vi "GetOtherStimulusArrayValues.vi"(3 "time between onset index":i32, 4 "fraction of time between index":i32, 5 "Cluster":cluster{"Value":sgl[][], "Value":i32[][]}, 6 "time since beginning of run":i32) -> (0 "time between onset index out":i32, 1 "fraction of time between index out":i32, 2 "stimulus settings":cluster{"outy3":sgl, "outy3":i32})   [LabVIEW 2015]
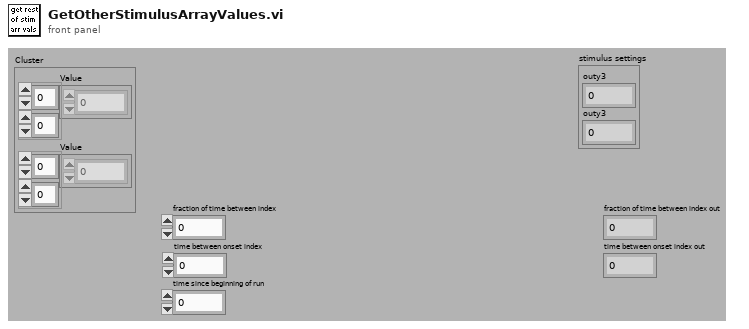
[diagram p1: front panel]
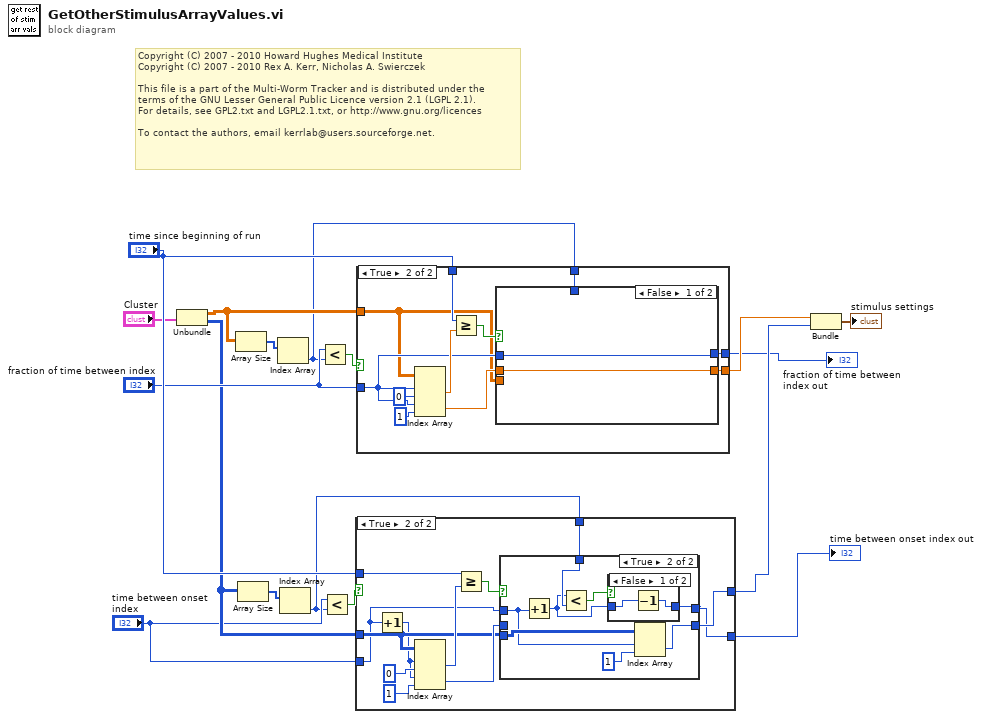
[diagram p0: block diagram]
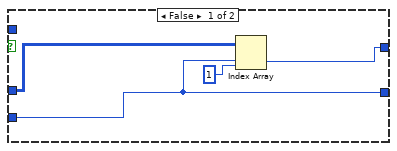
[diagram p2: hidden frame]
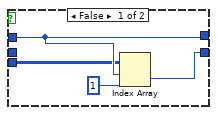
[diagram p3: hidden frame]
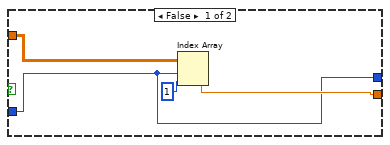
[diagram p5: hidden frame]
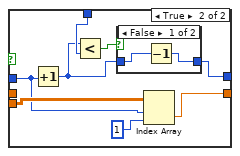
[diagram p6: hidden frame]
diagram:
  # "Copyright (C) 2007 - 2010 Howard Hughes Medical Institute\nCopyright (C) 2007 - 2010 Rex A. Kerr, Nicholas A. Swierczek\n \nThis file is a part of the Multi-Worm Tracker and is distributed under the\nterms of the GNU Lesser General Public Licence version 2.1 (LGPL 2.1).\nFor details, see GPL2.txt and LGPL2.1.txt, or http://www.gnu.org/licences\n \nTo contact the authors, email kerrlab@users.sourceforge.net."
  n1 = Unbundle("Cluster") -> ("Value"=w9:sgl[][], "Value"=w3:i32[][])
  n2 = Array Size(array=w9) -> (size(s)=w10:i32[])
  n3 = Array Size(array=w3) -> (size(s)=w5:i32[])
  n4 = Index Array(array=w10) -> (element=w6:i32)  [unwired: 1 in]
  n5 = Index Array(array=w5) -> (element=w1:i32)  [unwired: 1 in]
  n6 = Less?(x="fraction of time between index", y=w6) -> (x < y?=w8:bool)
  n7 = Less?(x="time between onset index", y=w1) -> (x < y?=w4:bool)
  n8 = case shown="True" w4 {
    tunnel: "time between onset index" -> [w18 w23]
    tunnel: [w19 w31] -> w16
    tunnel: "time since beginning of run" -> [_ w28]
    tunnel: w3 -> [w20 w26]
    tunnel: [w18 w25] -> w13
    tunnel: w1 -> [_ w24]
    frame False {
      n9 = Index Array(array=w20, index (row)=w18, index (col)=1 ("disabled index (col)")) -> (element=w19:i32)
    }
    frame True {
      n10 = Increment(x=w23) -> (x+1=w22:i32)
      n11 = Index Array(array=w26, index (row) #1=w22, index (col) #1=0 ("disabled index (col)"), index (row) #2=w22, index (col) #2=1 ("disabled index (col)")) -> (element #1=w29:i32, element #2=w27:i32)
      n12 = Greater Or Equal?(x=w28, y=w29) -> (x >= y?=w30:bool)
      n13 = case shown="True" w30 {
        tunnel: [w36 w43] -> w31
        tunnel: w27 -> [_ _]
        tunnel: w23 -> [w35 w42]
        tunnel: [w35 w39] -> w25
        tunnel: w26 -> [w34 w45]
        tunnel: w24 -> [_ w41]
        frame False {
          n14 = Index Array(array=w34, index (row)=w35, index (col)=1 ("disabled index (col)")) -> (element=w36:i32)
        }
        frame True {
          n15 = Increment(x=w42) -> (x+1=w38:i32)
          n16 = Less?(x=w38, y=w41) -> (x < y?=w40:bool)
          n17 = case shown="False" w40 {
            tunnel: [w46 w48] -> w39
            tunnel: w38 -> [w47 w48]
            frame False {
              n18 = Decrement(x=w47) -> (x-1=w46:i32)
            }
            frame True {
            }
          }
          n19 = Index Array(array=w45, index (row)=w42, index (col)=1 ("disabled index (col)")) -> (element=w43:i32)
        }
      }
    }
  }
  "time between onset index out" <- w13
  n20 = case shown="True" w8 {
    tunnel: [w51 w59] -> w17
    tunnel: "fraction of time between index" -> [w50 w57]
    tunnel: "time since beginning of run" -> [_ w56]
    tunnel: [w50 w55] -> w14
    tunnel: w9 -> [w52 w54]
    tunnel: w6 -> [_ w53]
    frame False {
      n21 = Index Array(array=w52, index (row)=w50, index (col)=1 ("disabled index (col)")) -> (element=w51:sgl)
    }
    frame True {
      n22 = Index Array(array=w54, index (row) #1=w57, index (col) #1=0 ("disabled index (col)"), index (row) #2=w57, index (col) #2=1 ("disabled index (col)")) -> (element #1=w63:sgl, element #2=w58:sgl)
      n23 = Greater Or Equal?(x=w56, y=w63) -> (x >= y?=w60:bool)
      n24 = case shown="False" w60 {
        tunnel: [w65 w71] -> w59
        tunnel: w58 -> [w65 _]
        tunnel: w57 -> [w64 w68]
        tunnel: [w64 w66] -> w55
        tunnel: w54 -> [_ w73]
        tunnel: w53 -> [_ w70]
        frame False {
        }
        frame True {
          n25 = Increment(x=w68) -> (x+1=w67:i32)
          n26 = Less?(x=w67, y=w70) -> (x < y?=w69:bool)
          n27 = case shown="False" w69 {
            tunnel: [w74 w76] -> w66
            tunnel: w67 -> [w75 w76]
            frame False {
              n28 = Decrement(x=w75) -> (x-1=w74:i32)
            }
            frame True {
            }
          }
          n29 = Index Array(array=w73, index (row)=w68, index (col)=1 ("disabled index (col)")) -> (element=w71:sgl)
        }
      }
    }
  }
  "fraction of time between index out" <- w14
  n30 = Bundle("outy3"=w17, "outy3"=w16) -> (→"stimulus settings":cluster{"outy3":sgl, "outy3":i32})  [unwired: 1 in]
